vi "Enqueue Guide_Light_Switch.vi"(8 "Error In":errorcluster, 10 "Light":bool, 11 "Name":string) -> (0 "Error Out":errorcluster, 2 "Data":variant)   [LabVIEW 2019, in "SR_2000.lvlib"]
uses:
  SR_2000.lvlib
  Queue/Queue.lvlib
  Data Error Notifier/Data and Error Notifier.lvlib
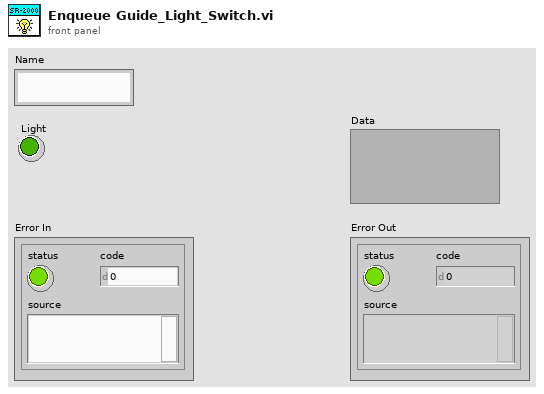
[diagram p1: front panel]
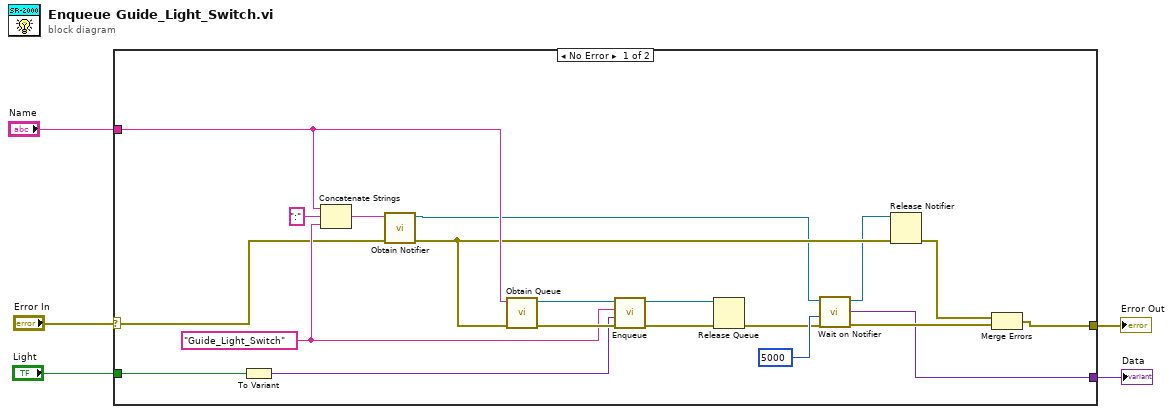
[diagram p0: block diagram]
diagram:
  n1 = case shown="No Error" "Error In" {
    selector: "Error In" -> [w13 w26]
    tunnel: [w17 w26] -> w4
    tunnel: "Name" -> [w24 _]
    tunnel: "Light" -> [w16 _]
    tunnel: [w6 _] -> w1
    frame No Error {
      w22 = "Guide_Light_Switch" ("Message")
      n2 = To Variant(anything=w16) -> (Variant=w15:variant)
      n3 = Concatenate Strings(w24, ":" ("string"), w22) -> (w14:string)
      n4 = call "Obtain Notifier.vi"("Error In"=w13, "Name"=w14) -> ("Error Out"=w12:errorcluster, "notifier out"=w11:refnum<notifier>)  [unwired: 8 in]
      n5 = call "Obtain Queue.vi"("Error In"=w12, "Name"=w24) -> ("Error Out"=w25:errorcluster, "queue out"=w20:refnum<queue>)  [unwired: 8 in]
      n6 = call "Enqueue.vi"("Error In"=w25, "Data"=w15, "Message"=w22, "queue in"=w20) -> ("Error Out"=w21:errorcluster, "queue out"=w19:refnum<queue>)  [unwired: 6 in]
      n7 = Release Queue(queue=w19, error in (no error)=w21) -> (error out=w9:errorcluster)  [unwired: 1 in, 2 out]
      n8 = call "Wait on Notifier.vi"("Error In"=w9, "timeout in ms (-1)"=5000, "notifier in"=w11) -> ("Error Out"=w7:errorcluster, "Data"=w6:variant, "notifier out"=w8:refnum<notifier>)  [unwired: 6 in]
      n9 = Release Notifier(notifier=w8, error in (no error)=w12) -> (error out=w18:errorcluster)  [unwired: 1 in, 2 out]
      n10 = Merge Errors(w18, w7) -> (w17:errorcluster)
    }
    frame Error {
    }
  }
  "Error Out" <- w4
  "Data" <- w1
